vi "Read Metrics.vi"(8 "error in (no error)":errorcluster, 11 "Registry Session in":refnum<class "Registry Session.lvclass">) -> (0 "error out":errorcluster, 2 "Metrics":map{string, refnum<data-value>}(c390), 3 "Registry Session out":refnum<class "Registry Session.lvclass">)   [LabVIEW 2020, in "Registry.lvlib" / "Registry Session.lvclass"]
uses:
  Registry Session.lvclass
  metrics/metric/Metric.lvclass
  Registry Session.lvclass/Registry Session.ctl
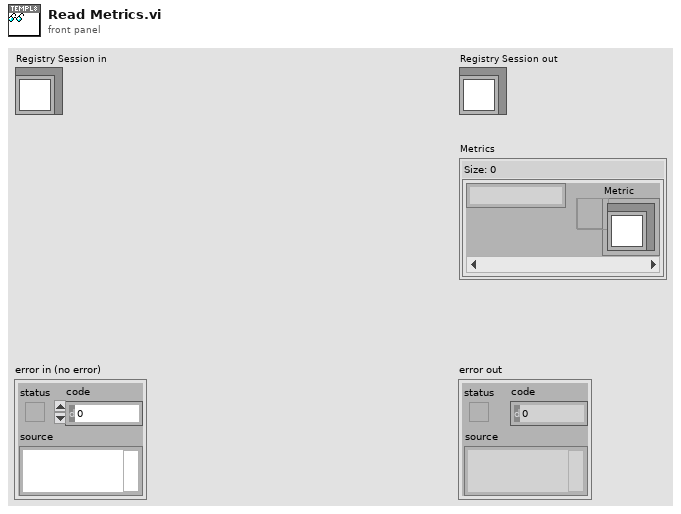
[diagram p1: front panel]
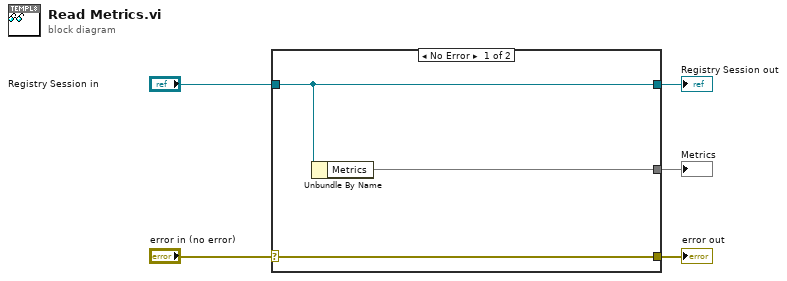
[diagram p0: block diagram]
diagram:
  n1 = case shown="No Error" "error in (no error)" {
    selector: "error in (no error)" -> [w8 w9]
    tunnel: [w8 w9] -> w4
    tunnel: [w7 w10] -> w2
    tunnel: "Registry Session in" -> [w7 w10]
    tunnel: [w6 _] -> w1
    frame No Error {
      n2 = Unbundle By Name(w7) -> ("Metrics"=w6:map{string, refnum<data-value>})
    }
    frame Error {
    }
  }
  "error out" <- w4
  "Registry Session out" <- w2
  "Metrics" <- w1
